vi "Read_Config.vi"(6 "configuration file path":path=path "/1699-preferences.ini") -> (1 "PID Out":T1, 2 "cluster":T2, 3 "cluster 2":T2, 4 "Array":string[][](array[string]))   [LabVIEW 2014]
uses:
  <vilib>/Utility/config.llb/Read Key (String).vi
  <vilib>/Utility/config.llb/NI_LVConfig.lvlib
panel:
  out "section":string
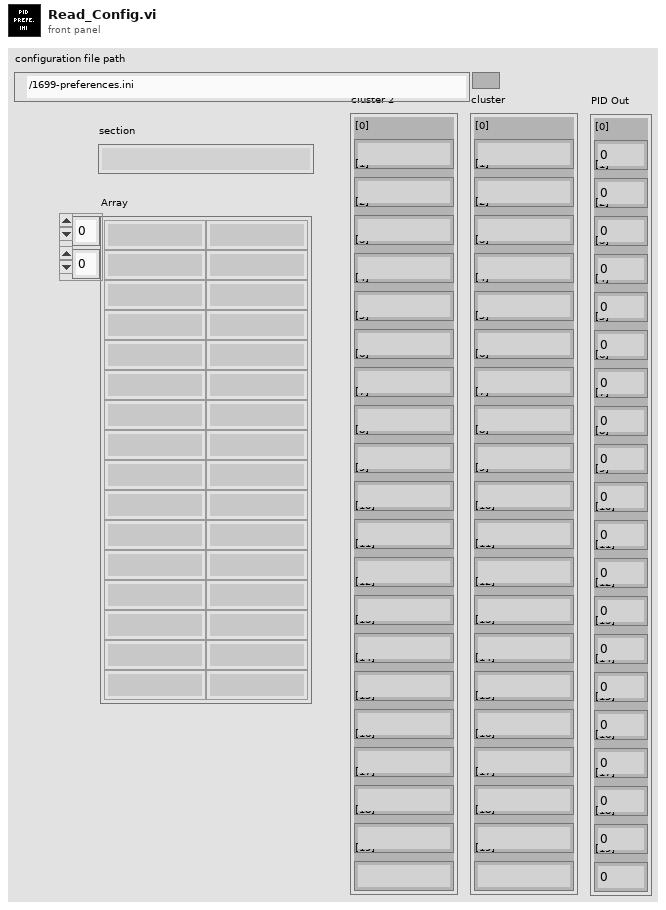
[diagram p1: front panel]
types:
  T1 = cluster{"[0]":dbl, "[1]":dbl, "[2]":dbl, "[3]":dbl, "[4]":dbl, "[5]":dbl, "[6]":dbl, "[7]":dbl, "[8]":dbl, "[9]":dbl, "[10]":dbl, "[11]":dbl, "[12]":dbl, "[13]":dbl, "[14]":dbl, "[15]":dbl, "[16]":dbl, "[17]":dbl, "[18]":dbl, "[19]":dbl}
  T2 = cluster{"[0]":string, "[1]":string, "[2]":string, "[3]":string, "[4]":string, "[5]":string, "[6]":string, "[7]":string, "[8]":string, "[9]":string, "[10]":string, "[11]":string, "[12]":string, "[13]":string, "[14]":string, "[15]":string, "[16]":string, "[17]":string, "[18]":string, "[19]":string}
  T3 = typedef "NI_LVConfig.lvlib/Config Data RefNum.ctl" = refnum<k1>
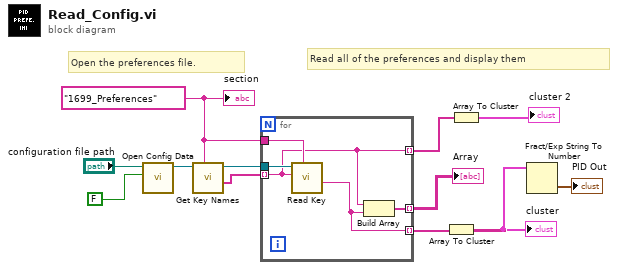
[diagram p0: block diagram]
diagram:
  w11 = "1699_Preferences" ("section")
  # "Read all of the preferences and display them"
  # "Open the preferences file."
  n1 = call <vilib>:"Open Config Data.vi"("create file if necessary (T)"=FALSE, "configuration file path"="configuration file path") -> ("refnum"=w9:T3)  [unwired: 7 in, 2 out]
  n2 = call <vilib>:"Get Key Names.vi"("section"=w11, "refnum"=w9) -> ("key names"=w10:string[], "refnum out"=w12:T3)  [unwired: 6 in, 2 out]
  n3 = for {
    tunnel: w10 -> [w13] mode=indexing
    tunnel: w12 -> [w17]
    tunnel: w11 -> [w16]
    tunnel: [w15] -> w8 mode=indexing
    tunnel: [w14] -> w7 mode=indexing
    tunnel: [w13] -> w6 mode=indexing
    n4 = call-poly <vilib>:"Read Key.vi"("section"=w16, "key"=w13, "refnum"=w17) -> ("value"=w14:string)  [unwired: 5 in, 3 out]
    n5 = Build Array(w13, w14) -> (w15:string[])
  }
  "Array" <- w8
  n6 = Array To Cluster(array=w7) -> (cluster=w4:T2)
  "cluster" <- w4
  n7 = Array To Cluster(array=w6) -> (cluster=→"cluster 2":T2)
  n8 = Fract/Exp String To Number(string=w4) -> (number=→"PID Out":T1)  [unwired: 3 in, 1 out]
  "section" <- w11
